vi "psychometric_function.vi"(7 "Response":bool, 8 "beta":dbl, 9 "T(i)":dbl, 10 "N":dbl[](array[numeric])) -> (3 "S(response, N)":dbl[](array[numeric]))   [LabVIEW 2022 SP3]
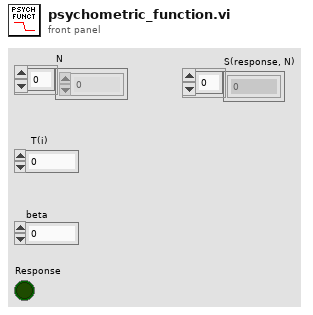
[diagram p1: front panel]
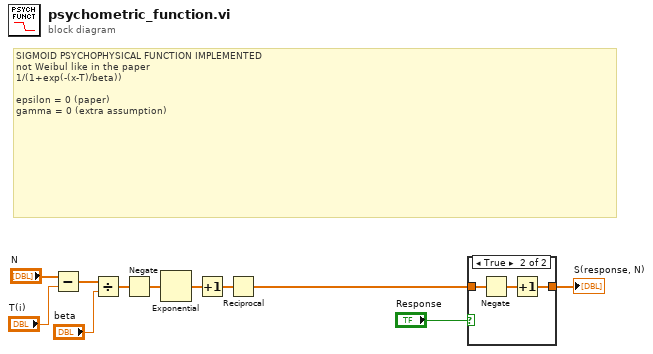
[diagram p0: block diagram]
diagram:
  # "SIGMOID PSYCHOPHYSICAL FUNCTION IMPLEMENTED\nnot Weibul like in the paper\n1/(1+exp(-(x-T)/beta))\n\nepsilon = 0 (paper)\ngamma = 0 (extra assumption)"
  n1 = Subtract(x="N", y="T(i)") -> (x-y=w9:dbl[])
  n2 = Divide(x=w9, y="beta") -> (x/y=w7:dbl[])
  n3 = Negate(x=w7) -> (-x=w6:dbl[])
  n4 = Exponential(1:w6) -> (0:w3:dbl[])
  n5 = Increment(x=w3) -> (x+1=w2:dbl[])
  n6 = Reciprocal(x=w2) -> (1/x=w5:dbl[])
  n7 = case shown="True" "Response" {
    tunnel: w5 -> [w12 w15]
    tunnel: [w12 w13] -> w1
    frame False {
    }
    frame True {
      n8 = Negate(x=w15) -> (-x=w14:dbl[])
      n9 = Increment(x=w14) -> (x+1=w13:dbl[])
    }
  }
  "S(response, N)" <- w1
